vi "COM emulator.vi"() -> ()   [LabVIEW 2021]
uses:
  <vilib>/Instr/_visa.llb/VISA Configure Serial Port (Instr).vi
panel:
  in  "Stop":bool
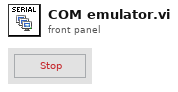
[diagram p1: front panel]
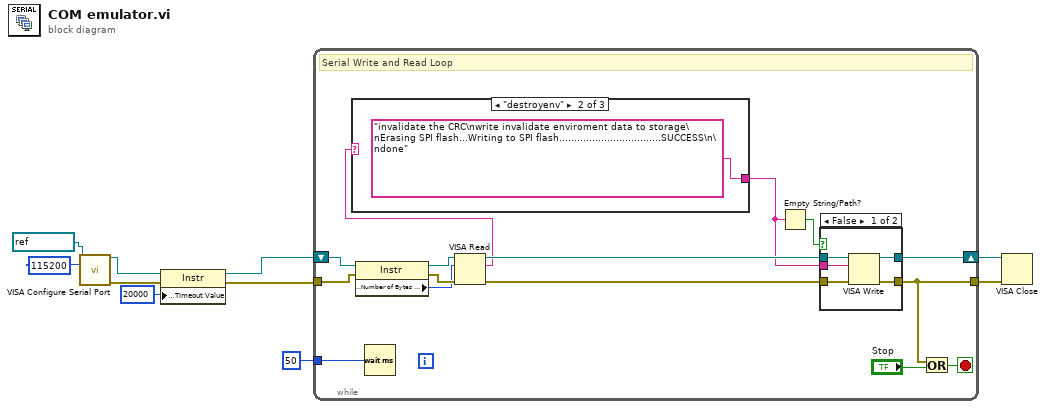
[diagram p0: block diagram]
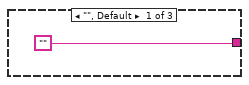
[diagram p3: hidden frame]
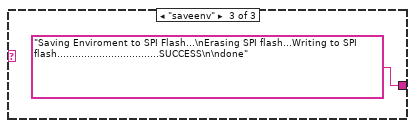
[diagram p4: hidden frame]
diagram:
  n1 = call-poly "VISA Configure Serial Port"("VISA resource name"=refnum<visa-resource-name> "COM2", "baud rate (9600)"=u32 115200) -> ("VISA resource name out"=w9:refnum<visa-resource-name>, "error out"=w8:errorcluster)  [unwired: 8 in, 4 out]
  n2 = property class="Instr"(reference=w9, error in=w8, "General Settings:Timeout Value"=u32 20000) -> (reference out=w4:refnum<visa-resource-name>, error out=w5:errorcluster)
  n3 = while {
    shift-right: [w21] -> w1
    shift-left: w4 -> [w13]
    tunnel: [w16] -> w2
    tunnel: w5 -> [w12]
    tunnel: u16 50 ("delay") -> [w24]
    stop <- w25 stop-if-true
    # "Serial Write and Read Loop"
    n4 = property class="Instr"(reference=w13, error in=w12) -> (reference out=w14:refnum<visa-resource-name>, error out=w15:errorcluster, "Serial Settings:Number of Bytes at Serial Port"=w11:u32)
    n5 = Wait (ms)(milliseconds to wait=w24) -> ()  [unwired: 1 out]
    n6 = VISA Read(VISA resource name=w14, byte count=w11, error in (no error)=w15) -> (VISA resource name out=w22:refnum<visa-resource-name>, read buffer=w20:string, error out=w17:errorcluster)  [unwired: 1 out]
    n7 = case shown="\"destroyenv\"" w20 {
      tunnel: ["" "invalidate the CRC\nwrite invalidate enviroment data to storage\nErasing SPI flash...Writing to SPI flash..................................SUCCESS\n\ndone" "Saving Enviroment to SPI Flash...\nErasing SPI flash...Writing to SPI flash..................................SUCCESS\n\ndone"] -> w18
      frame "", Default {
      }
      frame "destroyenv" {
      }
      frame "saveenv" {
      }
    }
    n8 = Empty String/Path?(string/path=w18) -> (empty?=w19:bool)
    n9 = case shown="False" w19 {
      tunnel: w22 -> [w30 w32]
      tunnel: [w29 w32] -> w21
      tunnel: w18 -> [w28 _]
      tunnel: w17 -> [w27 w31]
      tunnel: [w26 w31] -> w16
      frame False {
        n10 = VISA Write(VISA resource name=w30, write buffer=w28, error in (no error)=w27) -> (VISA resource name out=w29:refnum<visa-resource-name>, error out=w26:errorcluster)  [unwired: 1 out]
      }
      frame True {
      }
    }
    n11 = Or(x=w16, y="Stop") -> (x .or. y?=w25:bool)
  }
  n12 = VISA Close(VISA resource name=w1, error in (no error)=w2) -> ()  [unwired: 1 out]
